vi "main_panel.vi"() -> ()   [LabVIEW 2020]
uses:
  <vilib>/numeric/Random Number (Range) I64.vi
  <vilib>/numeric/sub_Random U32.vi
panel:
  out "Metoda Pardiso":dbl format="%#_6f"
  in  "?":bool=TRUE
  out "?":dbl[](array[numeric])
  in  "Liczba powtórzeń":i32=3
  in  "Tolerancja":ext=0.00001
  in  "Rozmiar macierzy":i32=100
  in  "Wybór układu":string(combo)="Diagonalnie Dominujący"
  in  "Wspólczynnik omega (SOR)":dbl=1.5 step=0.1
  out "?":dbl[](array[numeric])
  in  "?":bool=TRUE
  in  "?":bool=TRUE
  in  "?":bool=TRUE
  in  "?":bool=TRUE
  in  "?":bool=TRUE
  in  "?":bool=TRUE
  out "?":i32
  out "?":i32
  out "?":i32
  out "?":i32
  in  "?":dbl[](array[numeric])
  out "Wektor b":dbl[](array[numeric])
  out "Macierz A":dbl[][](array[numeric])
  in  "Rozwiązanie próbne x(0)":bool
  out "Metoda Gradientów Sprzężonych":dbl format="%#_6f"
  out "?":dbl[](array[numeric])
  out "Metoda Jacobiego":dbl format="%#_6f"
  out "?":dbl[](array[numeric])
  out "Metoda SOR":dbl format="%#_6f"
  out "?":dbl[](array[numeric])
  out "Metoda Gaussa-Seidla":dbl format="%#_6f"
  out "?":dbl[](array[numeric])
  out "Metoda  LU":dbl format="%#_6f"
  out "Metoda Wbudowana":dbl format="%#_7f"
  out "?":dbl[](array[numeric])
  # "Czas \nwykonania:"
  # "Czas \nwykonania:"
  # "Liczba iteracji:"
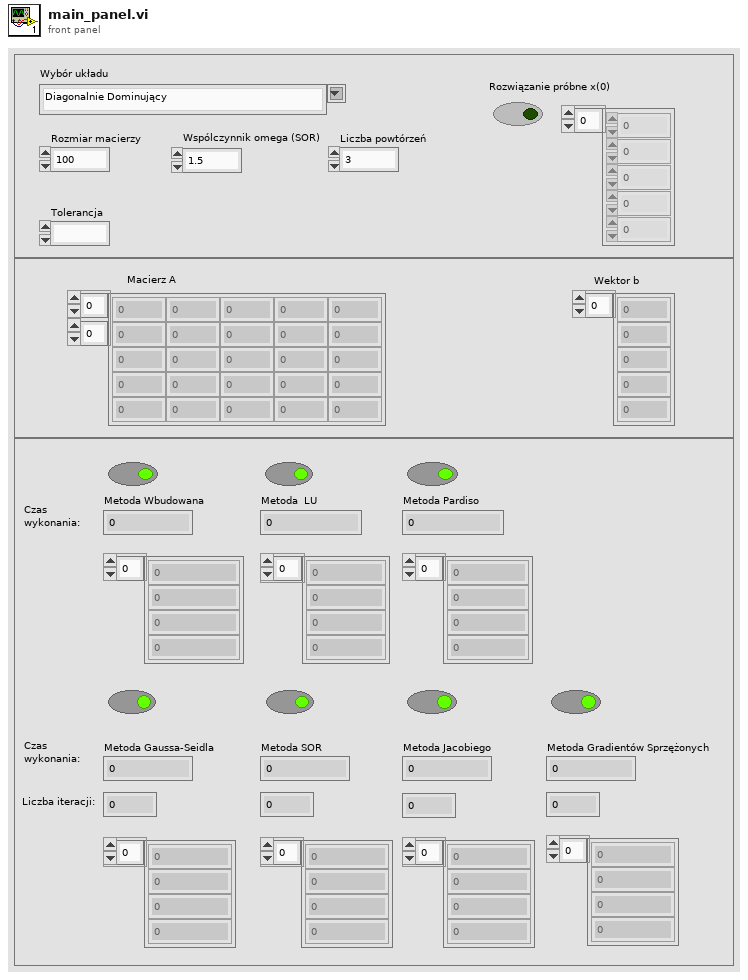
[diagram p1: front panel]
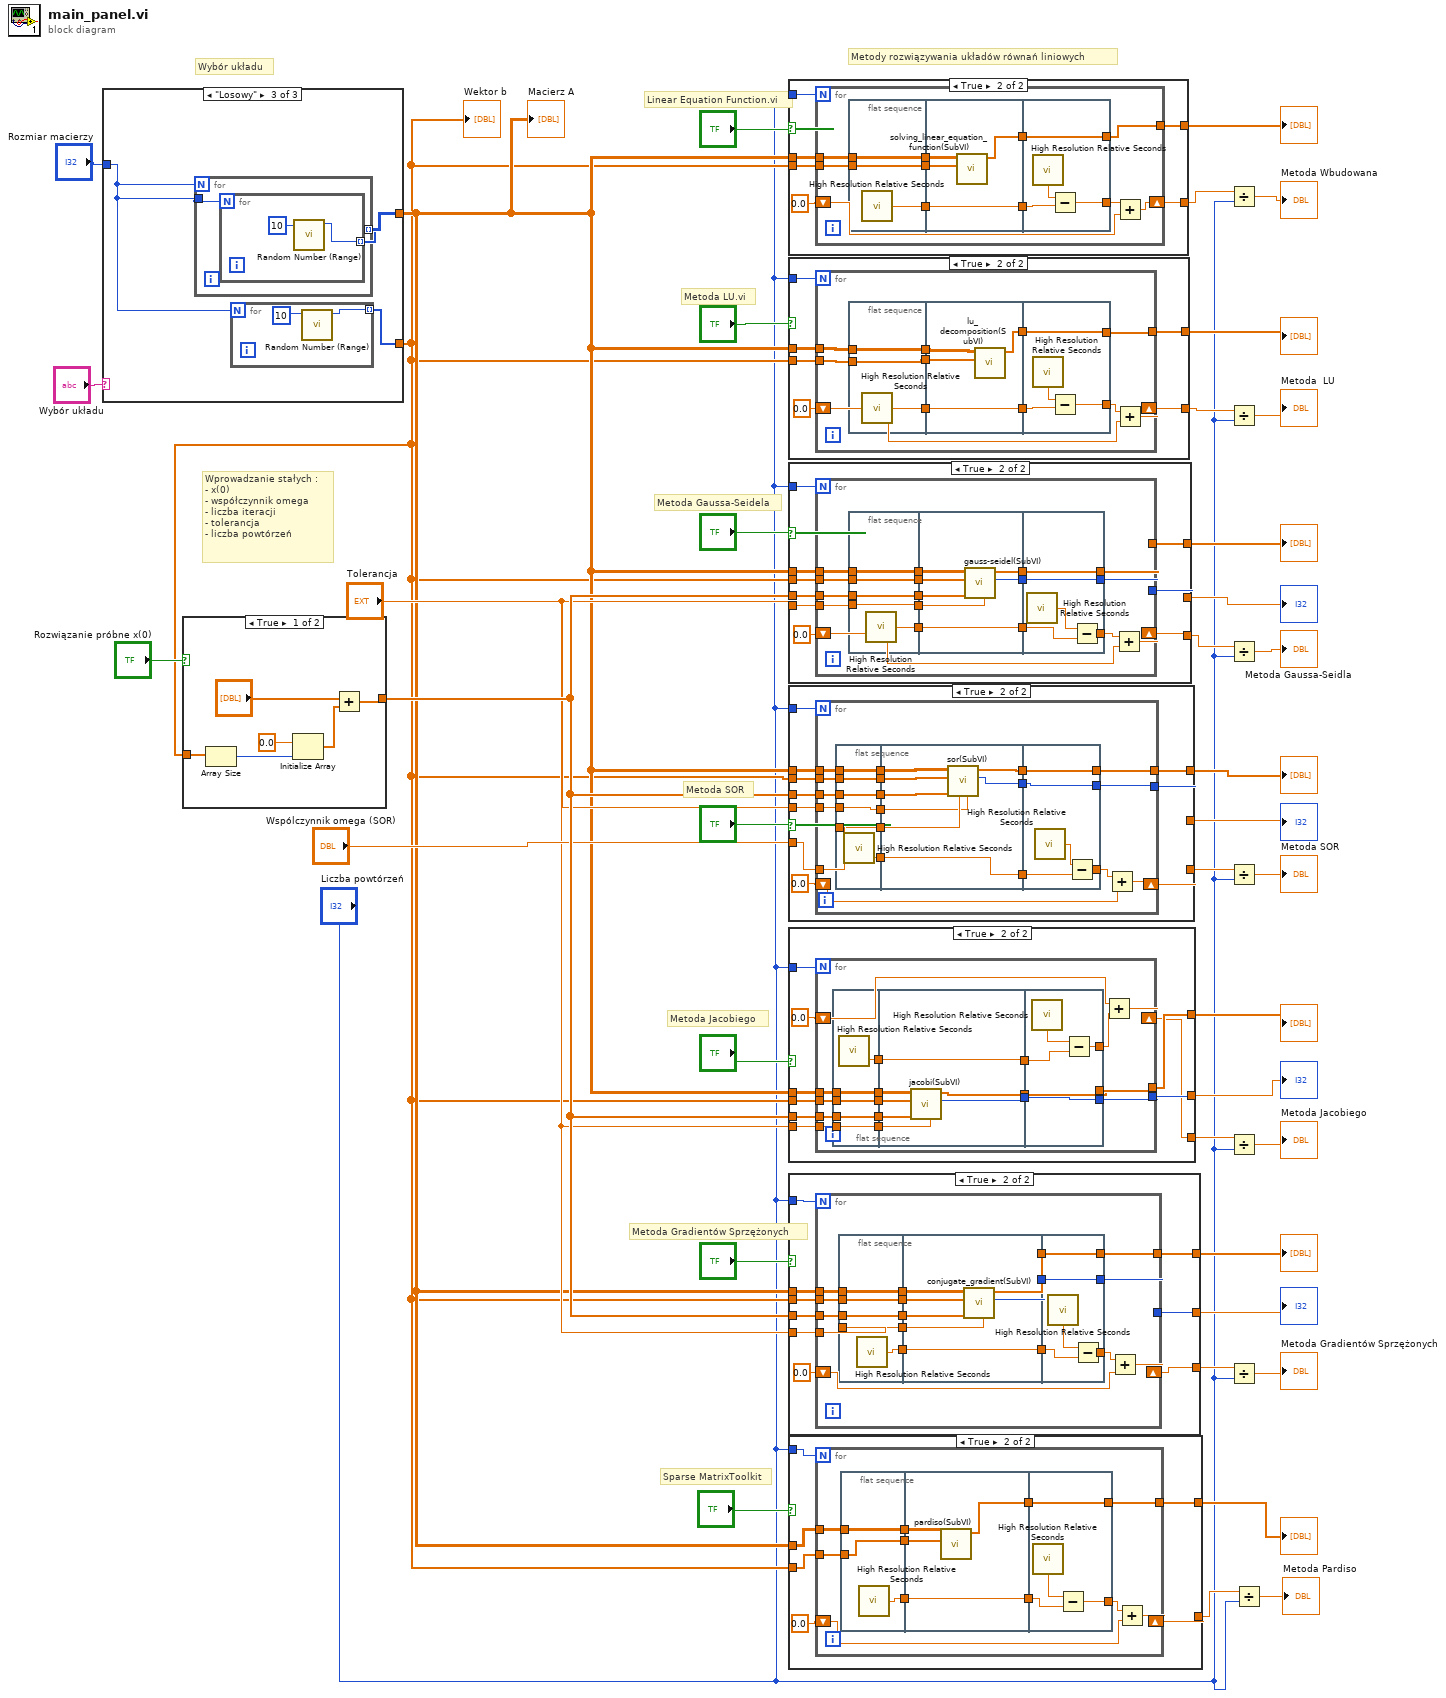
[diagram p0: block diagram]
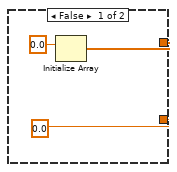
[diagram p2: hidden frame]
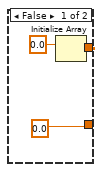
[diagram p3: hidden frame]
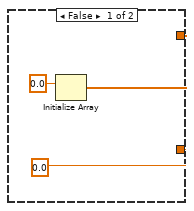
[diagram p4: hidden frame]
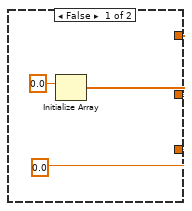
[diagram p5: hidden frame]
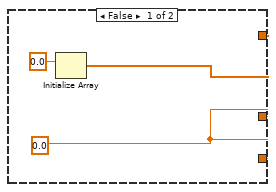
[diagram p6: hidden frame]
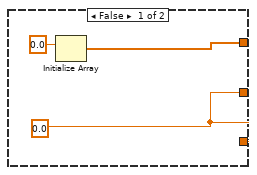
[diagram p7: hidden frame]
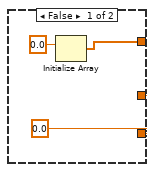
[diagram p8: hidden frame]
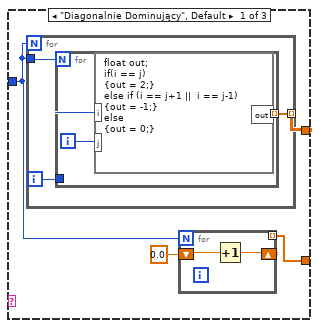
[diagram p9: hidden frame]
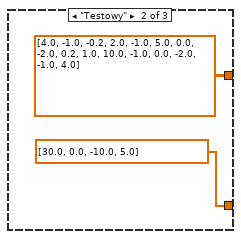
[diagram p10: hidden frame]
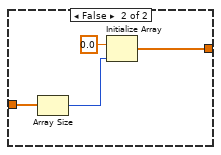
[diagram p11: hidden frame]
diagram:
  # "Sparse MatrixToolkit"
  # "Metoda Gradientów Sprzężonych"
  # "Metoda Jacobiego"
  # "Metoda SOR"
  # "Metoda Gaussa-Seidela"
  # "Metoda LU.vi"
  # "Linear Equation Function.vi"
  # "Wprowadzanie stałych : \n- x(0)\n- współczynnik omega\n- liczba iteracji\n- tolerancja\n- liczba powtórzeń"
  # "Wybór układu"
  # "Metody rozwiązywania układów równań liniowych"
  n1 = case shown="\"Losowy\"" "Wybór układu" {
    tunnel: "Rozmiar macierzy" -> [w45 _ w56]
    tunnel: [w42 dbl[] [30.0, 0.0, -10.0, 5.0] ("Array") w58] -> w2
    tunnel: [w43 dbl[][] [[4.0, -1.0, -0.2, 2.0], [-1.0, 5.0, 0.0, -2.0], [0.2, 1.0, 10.0, -1.0], [0.0, -2.0, -1.0, 4.0]] w57] -> w3
    frame "Diagonalnie Dominujący", Default {
      n2 = for {
        N: w45 -> [_]
        tunnel: w45 -> [w49]
        tunnel: [w48] -> w43 mode=indexing
        i -> [w50]
        n3 = for {
          N: w49 -> [_]
          tunnel: w50 -> [w53]
          tunnel: [w51] -> w48 mode=indexing
          i -> [w52]
          n4 = formula code="float out;\nif(i == j)\n{out = 2;}\nelse if (i == j+1 ||  i == j-1)\n{out = -1;}\nelse \n{out = 0;}"("i"=w53, "j"=w52) -> ("out"=w51:dbl)
        }
      }
      n5 = for {
        N: w45 -> [_]
        shift-right: [w47] -> _
        shift-left: 0.0 -> [w46]
        tunnel: [w47] -> w42 mode=indexing
        n6 = Increment(x=w46) -> (x+1=w47:dbl)
      }
    }
    frame "Testowy" {
    }
    frame "Losowy" {
      n7 = for {
        N: w56 -> [_]
        tunnel: [w60] -> w57 mode=indexing
        tunnel: w56 -> [w59]
        n8 = for {
          N: w59 -> [_]
          tunnel: [w62] -> w60 mode=indexing
          n9 = call-poly <vilib>:"Random Number (Range).vi"("upper bound (100)"=10) -> ("number"=w62:i64)  [unwired: 10 in]
        }
      }
      n10 = for {
        N: w56 -> [_]
        tunnel: [w64] -> w58 mode=indexing
        n11 = call-poly <vilib>:"Random Number (Range).vi"("upper bound (100)"=10) -> ("number"=w64:i64)  [unwired: 10 in]
      }
    }
  }
  "Macierz A" <- w3
  "Wektor b" <- w2
  n12 = case shown="True" "Rozwiązanie próbne x(0)" {
    tunnel: w2 -> [w65 w73]
    tunnel: [w66 w71] -> w35
    frame True {
      n13 = Array Size(array=w65) -> (size(s)=w70:i32)
      n14 = Initialize Array(0.0 ("element"), w70) -> (w68:dbl[])
      n15 = Add(x="?", y=w68) -> (x+y=w66:dbl[])
    }
    frame False {
      n16 = Array Size(array=w73) -> (size(s)=w72:i32)
      n17 = Initialize Array(0.0 ("element"), w72) -> (w71:dbl[])
    }
  }
  n18 = case shown="True" "?" {
    tunnel: w3 -> [_ w83]
    tunnel: w2 -> [_ w82]
    tunnel: [0.0 ("element") w81] -> w10
    tunnel: [w77 w80] -> w27
    tunnel: "Liczba powtórzeń" -> [_ w79]
    frame False {
      n19 = Initialize Array(0.0 ("element")) -> (w77:dbl[])  [unwired: 1 in]
    }
    frame True {
      n20 = for {
        N: w79 -> [_]
        tunnel: w83 -> [w89]
        tunnel: w82 -> [w88]
        tunnel: [w87] -> w80
        shift-right: [w85] -> w81
        shift-left: 0.0 -> [w84]
        n21 = flat-sequence {
          tunnel: w88 -> [w96]
          tunnel: w89 -> [w97]
          tunnel: [w97] -> w94
          tunnel: [w96] -> w93
          tunnel: [w95] -> w92
          tunnel: w94 -> [w101]
          tunnel: w93 -> [w100]
          tunnel: [w99] -> w91
          tunnel: w92 -> [w99]
          tunnel: [w98] -> w90
          tunnel: w91 -> [w105]
          tunnel: [w103] -> w86
          tunnel: [w102] -> w87
          tunnel: w90 -> [w102]
          frame #0 {
            n22 = call <vilib>:"High Resolution Relative Seconds.vi"() -> ("relative seconds"=w95:dbl)
          }
          frame #1 {
            n23 = call "solving_linear_equation_function(SubVI).vi"("Wektor b"=w100, "Macierz A"=w101) -> ("Wynik"=w98:dbl[])  [unwired: 9 in]
          }
          frame #2 {
            n24 = call <vilib>:"High Resolution Relative Seconds.vi"() -> ("relative seconds"=w104:dbl)
            n25 = Subtract(x=w104, y=w105) -> (x-y=w103:dbl)
          }
        }
        n26 = Add(x=w86, y=w84) -> (x+y=w85:dbl)
      }
    }
  }
  "?" <- w27
  n27 = case shown="True" "?" {
    tunnel: [0.0 ("element") w114] -> w9
    tunnel: [w107 w113] -> w38
    tunnel: w3 -> [_ w112]
    tunnel: w2 -> [_ w111]
    tunnel: "Liczba powtórzeń" -> [_ w110]
    frame False {
      n28 = Initialize Array(0.0 ("element")) -> (w107:dbl[])  [unwired: 1 in]
    }
    frame True {
      n29 = for {
        N: w110 -> [_]
        tunnel: [w120] -> w113
        tunnel: w112 -> [w119]
        tunnel: w111 -> [w118]
        shift-right: [w116] -> w114
        shift-left: 0.0 -> [w115]
        n30 = flat-sequence {
          tunnel: [w128] -> w125
          tunnel: w119 -> [w127]
          tunnel: [w127] -> w124
          tunnel: w118 -> [w126]
          tunnel: [w126] -> w123
          tunnel: [w132] -> w122
          tunnel: w125 -> [w132]
          tunnel: w124 -> [w131]
          tunnel: w123 -> [w130]
          tunnel: [w129] -> w121
          tunnel: w122 -> [w136]
          tunnel: [w134] -> w117
          tunnel: [w133] -> w120
          tunnel: w121 -> [w133]
          frame #0 {
            n31 = call <vilib>:"High Resolution Relative Seconds.vi"() -> ("relative seconds"=w128:dbl)
          }
          frame #1 {
            n32 = call "lu_decomposition(SubVI).vi"("Wektor b"=w130, "Macierz A"=w131) -> ("Wynik"=w129:dbl[])  [unwired: 9 in]
          }
          frame #2 {
            n33 = call <vilib>:"High Resolution Relative Seconds.vi"() -> ("relative seconds"=w135:dbl)
            n34 = Subtract(x=w135, y=w136) -> (x-y=w134:dbl)
          }
        }
        n35 = Add(x=w117, y=w115) -> (x+y=w116:dbl)
      }
    }
  }
  "?" <- w38
  n36 = case shown="True" "?" {
    tunnel: [w137 w148] -> w8
    tunnel: [w138 w147] -> w37
    tunnel: [w137 w146] -> w36
    tunnel: w35 -> [_ w145]
    tunnel: w3 -> [_ w144]
    tunnel: w2 -> [_ w143]
    tunnel: "Tolerancja" -> [_ w142]
    tunnel: "Liczba powtórzeń" -> [_ w141]
    frame False {
      w137 = 0.0 ("element")
      n37 = Initialize Array(0.0 ("element")) -> (w138:dbl[])  [unwired: 1 in]
    }
    frame True {
      n38 = for {
        N: w141 -> [_]
        tunnel: [w157] -> w147
        tunnel: w145 -> [w155]
        tunnel: w144 -> [w154]
        tunnel: w143 -> [w153]
        tunnel: w142 -> [w152]
        shift-right: [w150] -> w148
        shift-left: 0.0 -> [w149]
        tunnel: [w156] -> w146
        n39 = flat-sequence {
          tunnel: w153 -> [w168]
          tunnel: w154 -> [w169]
          tunnel: w155 -> [w170]
          tunnel: [w170] -> w165
          tunnel: [w169] -> w164
          tunnel: [w168] -> w163
          tunnel: [w167] -> w162
          tunnel: w152 -> [w166]
          tunnel: [w166] -> w161
          tunnel: w165 -> [w177]
          tunnel: w164 -> [w176]
          tunnel: w163 -> [w175]
          tunnel: [w174] -> w160
          tunnel: w162 -> [w174]
          tunnel: [w173] -> w159
          tunnel: [w172] -> w158
          tunnel: w161 -> [w171]
          tunnel: w160 -> [w181]
          tunnel: [w180] -> w151
          tunnel: w159 -> [w179]
          tunnel: [w179] -> w157
          tunnel: w158 -> [w178]
          tunnel: [w178] -> w156
          frame #0 {
            n40 = call <vilib>:"High Resolution Relative Seconds.vi"() -> ("relative seconds"=w167:dbl)
          }
          frame #1 {
            n41 = call "gauss-seidel(SubVI).vi"("Tolerancja"=w171, "Initial Guess"=w177, "Wektor b"=w175, "Macierz A"=w176) -> ("Wykonana iczba Iteracji"=w172:i32, "Metoda Gaussa-Seidla"=w173:dbl[])  [unwired: 6 in]
          }
          frame #2 {
            n42 = call <vilib>:"High Resolution Relative Seconds.vi"() -> ("relative seconds"=w182:dbl)
            n43 = Subtract(x=w182, y=w181) -> (x-y=w180:dbl)
          }
        }
        n44 = Add(x=w151, y=w149) -> (x+y=w150:dbl)
      }
    }
  }
  "?" <- w37
  "?" <- w36
  n45 = case shown="True" "?" {
    tunnel: w35 -> [_ w195]
    tunnel: [w183 w194] -> w15
    tunnel: "Wspólczynnik omega (SOR)" -> [_ w193]
    tunnel: [w184 w192] -> w33
    tunnel: [w183 w191] -> w32
    tunnel: w3 -> [_ w190]
    tunnel: w2 -> [_ w189]
    tunnel: "Tolerancja" -> [_ w188]
    tunnel: "Liczba powtórzeń" -> [_ w187]
    frame False {
      w183 = 0.0 ("element")
      n46 = Initialize Array(0.0 ("element")) -> (w184:dbl[])  [unwired: 1 in]
    }
    frame True {
      n47 = for {
        N: w187 -> [_]
        tunnel: w195 -> [w205]
        tunnel: [w203] -> w192
        tunnel: w190 -> [w201]
        tunnel: w189 -> [w200]
        tunnel: w188 -> [w199]
        tunnel: w193 -> [w204]
        tunnel: [w202] -> w191
        shift-right: [w197] -> w194
        shift-left: 0.0 -> [w196]
        n48 = flat-sequence {
          tunnel: w205 -> [w218]
          tunnel: w200 -> [w219]
          tunnel: w201 -> [w220]
          tunnel: [w220] -> w214
          tunnel: [w219] -> w213
          tunnel: [w218] -> w212
          tunnel: [w217] -> w211
          tunnel: w204 -> [w216]
          tunnel: [w216] -> w210
          tunnel: w199 -> [w215]
          tunnel: [w215] -> w209
          tunnel: w214 -> [w228]
          tunnel: w213 -> [w227]
          tunnel: w212 -> [w226]
          tunnel: [w225] -> w208
          tunnel: w211 -> [w225]
          tunnel: w210 -> [w224]
          tunnel: [w223] -> w207
          tunnel: [w222] -> w206
          tunnel: w209 -> [w221]
          tunnel: w208 -> [w233]
          tunnel: [w231] -> w198
          tunnel: w207 -> [w230]
          tunnel: [w230] -> w203
          tunnel: w206 -> [w229]
          tunnel: [w229] -> w202
          frame #0 {
            n49 = call <vilib>:"High Resolution Relative Seconds.vi"() -> ("relative seconds"=w217:dbl)
          }
          frame #1 {
            n50 = call "sor(SubVI).vi"("Tolerancja"=w221, "omega"=w224, "Initial Guess"=w226, "Macierz b"=w227, "Macierz A"=w228) -> ("Wykonana iczba Iteracji"=w222:i32, "Metoda SOR"=w223:dbl[])  [unwired: 5 in]
          }
          frame #2 {
            n51 = call <vilib>:"High Resolution Relative Seconds.vi"() -> ("relative seconds"=w232:dbl)
            n52 = Subtract(x=w232, y=w233) -> (x-y=w231:dbl)
          }
        }
        n53 = Add(x=w198, y=w196) -> (x+y=w197:dbl)
      }
    }
  }
  "?" <- w33
  "?" <- w32
  n54 = case shown="True" "?" {
    tunnel: w35 -> [_ w245]
    tunnel: [w234 w238] -> w17
    tunnel: [w235 w244] -> w31
    tunnel: [w234 w243] -> w30
    tunnel: w3 -> [_ w242]
    tunnel: w2 -> [_ w241]
    tunnel: "Tolerancja" -> [_ w240]
    tunnel: "Liczba powtórzeń" -> [_ w239]
    frame False {
      w234 = 0.0 ("element")
      n55 = Initialize Array(0.0 ("element")) -> (w235:dbl[])  [unwired: 1 in]
    }
    frame True {
      n56 = for {
        N: w239 -> [_]
        tunnel: w245 -> [w254]
        tunnel: [w253] -> w244
        tunnel: w242 -> [w251]
        tunnel: w241 -> [w250]
        tunnel: w240 -> [w249]
        tunnel: [w252] -> w243
        shift-right: [w246] -> w238
        shift-left: 0.0 -> [w247]
        n57 = flat-sequence {
          tunnel: w254 -> [w265]
          tunnel: w250 -> [w266]
          tunnel: w251 -> [w267]
          tunnel: [w267] -> w262
          tunnel: [w266] -> w261
          tunnel: [w265] -> w260
          tunnel: [w264] -> w259
          tunnel: w249 -> [w263]
          tunnel: [w263] -> w258
          tunnel: w262 -> [w274]
          tunnel: w261 -> [w273]
          tunnel: w260 -> [w272]
          tunnel: [w271] -> w257
          tunnel: w259 -> [w271]
          tunnel: [w270] -> w256
          tunnel: [w269] -> w255
          tunnel: w258 -> [w268]
          tunnel: w257 -> [w278]
          tunnel: [w277] -> w248
          tunnel: [w276] -> w253
          tunnel: w256 -> [w276]
          tunnel: w255 -> [w275]
          tunnel: [w275] -> w252
          frame #0 {
            n58 = call <vilib>:"High Resolution Relative Seconds.vi"() -> ("relative seconds"=w264:dbl)
          }
          frame #1 {
            n59 = call "jacobi(SubVI).vi"("Tolerancja"=w268, "Initiial Guess"=w272, "b"=w273, "A"=w274) -> ("Wykonana iczba Iteracji"=w269:i32, "Metoda Jacobiego"=w270:dbl[])  [unwired: 6 in]
          }
          frame #2 {
            n60 = call <vilib>:"High Resolution Relative Seconds.vi"() -> ("relative seconds"=w279:dbl)
            n61 = Subtract(x=w279, y=w278) -> (x-y=w277:dbl)
          }
        }
        n62 = Add(x=w247, y=w248) -> (x+y=w246:dbl)
      }
    }
  }
  "?" <- w31
  "?" <- w30
  n63 = case shown="True" "?" {
    tunnel: w35 -> [_ w291]
    tunnel: [w280 w290] -> w19
    tunnel: [w281 w289] -> w21
    tunnel: [w280 w288] -> w29
    tunnel: w3 -> [_ w287]
    tunnel: w2 -> [_ w286]
    tunnel: "Tolerancja" -> [_ w285]
    tunnel: "Liczba powtórzeń" -> [_ w284]
    frame False {
      w280 = 0.0 ("element")
      n64 = Initialize Array(0.0 ("element")) -> (w281:dbl[])  [unwired: 1 in]
    }
    frame True {
      n65 = for {
        N: w284 -> [_]
        tunnel: w291 -> [w300]
        tunnel: [w299] -> w289
        tunnel: w287 -> [w297]
        tunnel: w286 -> [w296]
        tunnel: w285 -> [w295]
        tunnel: [w298] -> w288
        shift-right: [w293] -> w290
        shift-left: 0.0 -> [w292]
        n66 = flat-sequence {
          tunnel: w300 -> [w311]
          tunnel: w296 -> [w312]
          tunnel: w297 -> [w313]
          tunnel: [w313] -> w308
          tunnel: [w312] -> w307
          tunnel: [w311] -> w306
          tunnel: [w310] -> w305
          tunnel: [w309] -> w304
          tunnel: w295 -> [w309]
          tunnel: w308 -> [w320]
          tunnel: w307 -> [w319]
          tunnel: w306 -> [w318]
          tunnel: w305 -> [w317]
          tunnel: [w317] -> w303
          tunnel: [w316] -> w302
          tunnel: [w315] -> w301
          tunnel: w304 -> [w314]
          tunnel: w303 -> [w324]
          tunnel: [w323] -> w294
          tunnel: w302 -> [w322]
          tunnel: [w322] -> w299
          tunnel: w301 -> [w321]
          tunnel: [w321] -> w298
          frame #0 {
            n67 = call <vilib>:"High Resolution Relative Seconds.vi"() -> ("relative seconds"=w310:dbl)
          }
          frame #1 {
            n68 = call "conjugate_gradient(SubVI).vi"("Tolerancja"=w314, "Initial Guess"=w318, "b"=w319, "A"=w320) -> ("Wykonana iczba Iteracji"=w315:i32, "Gradientów Sprzężonych"=w316:dbl[])  [unwired: 6 in]
          }
          frame #2 {
            n69 = call <vilib>:"High Resolution Relative Seconds.vi"() -> ("relative seconds"=w325:dbl)
            n70 = Subtract(x=w325, y=w324) -> (x-y=w323:dbl)
          }
        }
        n71 = Add(x=w294, y=w292) -> (x+y=w293:dbl)
      }
    }
  }
  "?" <- w29
  "?" <- w21
  n72 = case shown="True" "?" {
    tunnel: [0.0 ("element") w334] -> w5
    tunnel: [w327 w333] -> w7
    tunnel: "Liczba powtórzeń" -> [_ w332]
    tunnel: w3 -> [_ w330]
    tunnel: w2 -> [_ w329]
    frame False {
      n73 = Initialize Array(0.0 ("element")) -> (w327:dbl[])  [unwired: 1 in]
    }
    frame True {
      n74 = for {
        N: w332 -> [_]
        tunnel: [w342] -> w333
        shift-right: [w340] -> w334
        shift-left: 0.0 -> [w339]
        tunnel: w330 -> [w338]
        tunnel: w329 -> [w336]
        n75 = flat-sequence {
          tunnel: [w348] -> w345
          tunnel: w338 -> [w347]
          tunnel: [w347] -> w337
          tunnel: w336 -> [w346]
          tunnel: [w346] -> w335
          tunnel: w345 -> [w352]
          tunnel: [w352] -> w344
          tunnel: [w349] -> w343
          tunnel: w337 -> [w351]
          tunnel: w335 -> [w350]
          tunnel: w344 -> [w355]
          tunnel: [w354] -> w341
          tunnel: w343 -> [w353]
          tunnel: [w353] -> w342
          frame #0 {
            n76 = call <vilib>:"High Resolution Relative Seconds.vi"() -> ("relative seconds"=w348:dbl)
          }
          frame #1 {
            n77 = call "pardiso(SubVI).vi"("b"=w350, "A"=w351) -> ("Wynik"=w349:dbl[])  [unwired: 9 in]
          }
          frame #2 {
            n78 = call <vilib>:"High Resolution Relative Seconds.vi"() -> ("relative seconds"=w356:dbl)
            n79 = Subtract(x=w356, y=w355) -> (x-y=w354:dbl)
          }
        }
        n80 = Add(x=w341, y=w339) -> (x+y=w340:dbl)
      }
    }
  }
  "?" <- w7
  n81 = Divide(x=w10, y="Liczba powtórzeń") -> (x/y=→"Metoda Wbudowana":dbl)
  n82 = Divide(x=w9, y="Liczba powtórzeń") -> (x/y=→"Metoda  LU":dbl)
  n83 = Divide(x=w8, y="Liczba powtórzeń") -> (x/y=→"Metoda Gaussa-Seidla":dbl)
  n84 = Divide(x=w15, y="Liczba powtórzeń") -> (x/y=→"Metoda SOR":dbl)
  n85 = Divide(x=w17, y="Liczba powtórzeń") -> (x/y=→"Metoda Jacobiego":dbl)
  n86 = Divide(x=w19, y="Liczba powtórzeń") -> (x/y=→"Metoda Gradientów Sprzężonych":dbl)
  n87 = Divide(x=w5, y="Liczba powtórzeń") -> (x/y=→"Metoda Pardiso":dbl)
